vi "initImageAll.vi"() -> (3 "Refnum out":T1)   [LabVIEW 2013, in "MagAnalysis_Online.lvclass"]
uses:
  MagAnalysis_Online.lvclass
  <vilib>/vision/Image Controls.llb/IMAQ Image.ctl
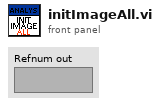
[diagram p1: front panel]
types:
  T1 = typedef "IMAQ Image.ctl" = refnum<image>
  T2 = typedef "Image Type" = u32
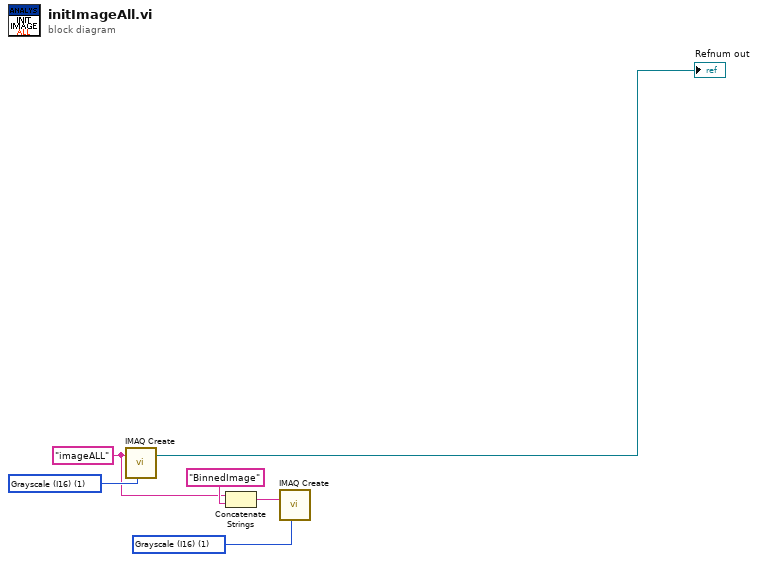
[diagram p0: block diagram]
diagram:
  w1 = T2 1 items=["Grayscale (U8)", "Grayscale (I16)", "Grayscale (SGL)", "Complex (CSG)", "RGB (U32)", "HSL (U32)", "RGB (U64)", "Grayscale (U16)"] ("Image Type")
  w6 = T2 1 items=["Grayscale (U8)", "Grayscale (I16)", "Grayscale (SGL)", "Complex (CSG)", "RGB (U32)", "HSL (U32)", "RGB (U64)", "Grayscale (U16)"] ("Image Type")
  w3 = "imageALL" ("Image Name")
  n1 = call "IMAQ Create"("Image Name"=w3, "Image Type"=w6) -> ("New Image"=→"Refnum out":T1)  [unwired: 3 in, 1 out]
  n2 = Concatenate Strings(w3, "BinnedImage") -> (w5:string)
  n3 = call "IMAQ Create"("Image Name"=w5, "Image Type"=w1) -> ()  [unwired: 3 in, 2 out]
